vi "DataWaveformChart.vi"(9 "FFT full energy":dbl, 10 "timestamp":dbl, 11 "waveform chart":refnum<vi>) -> ()   [LabVIEW 2018, in "statistics.lvlib"]
uses:
  statistics.lvlib
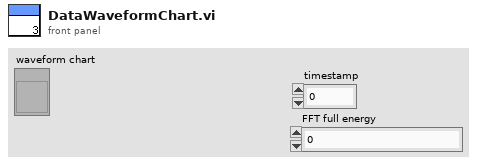
[diagram p1: front panel]
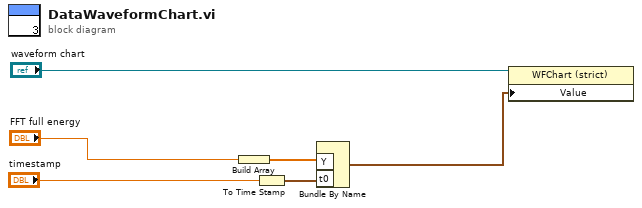
[diagram p0: block diagram]
diagram:
  n1 = Build Array("FFT full energy") -> (w4:dbl[])
  n2 = To Time Stamp(1:"timestamp") -> (0:w6:timestamp)
  n3 = Bundle By Name("Y"=w4, "t0"=w6) -> (w1:waveform(dbl))  [unwired: 1 in]
  n4 = property class="WFChart (strict)"(reference="waveform chart", "Value"=w1) -> ()  [unwired: 1 in, 2 out]
